vi "test_ssh.vi"(5 "Close?":bool=TRUE, 7 "Connection Info.":T2={"Remote"="10.8.2.13", "Username"="tvt", "Port (22)"=22}, 8 "error in (no error)":errorcluster, 9 "Delay Time (s)":dbl=10.0 format="%#_13g", 11 "cmd Box":string(combo)) -> (0 "error out":errorcluster, 2 "cmd string":string, 3 "remote log path":string)   [LabVIEW 2022 SP3]
uses:
  SSH Library/Connection Info..cluster.ctl
  SSH Library/Password..cluster.ctl
  <vilib>/Utility/error.llb/Trim Whitespace One-Sided.vi
  SSH Library/connect_password.vi
  SSH Library/LabSSH.lvlib
panel:
  out "Connection Name":string
  out "Method Response":string
  out "isSshConnected":bool
  in  "Password":T1={"Password"="TDDPc5kc4WnYcy"}
  out "Output":string
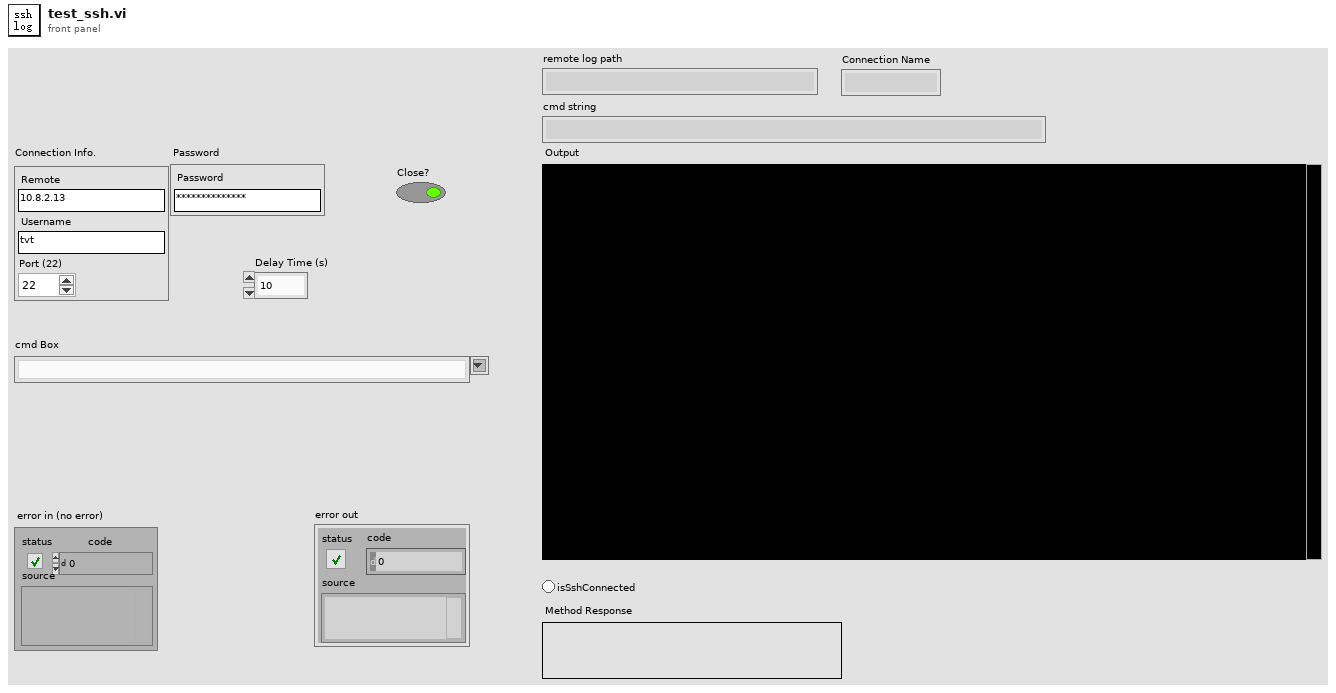
[diagram p1: front panel]
types:
  T1 = typedef "LabSSH.lvlib/Password..cluster.ctl" = cluster{"Password":string}
  T2 = typedef "LabSSH.lvlib/Connection Info..cluster.ctl" = cluster{"Remote":string, "Username":string, "Port (22)":i32}
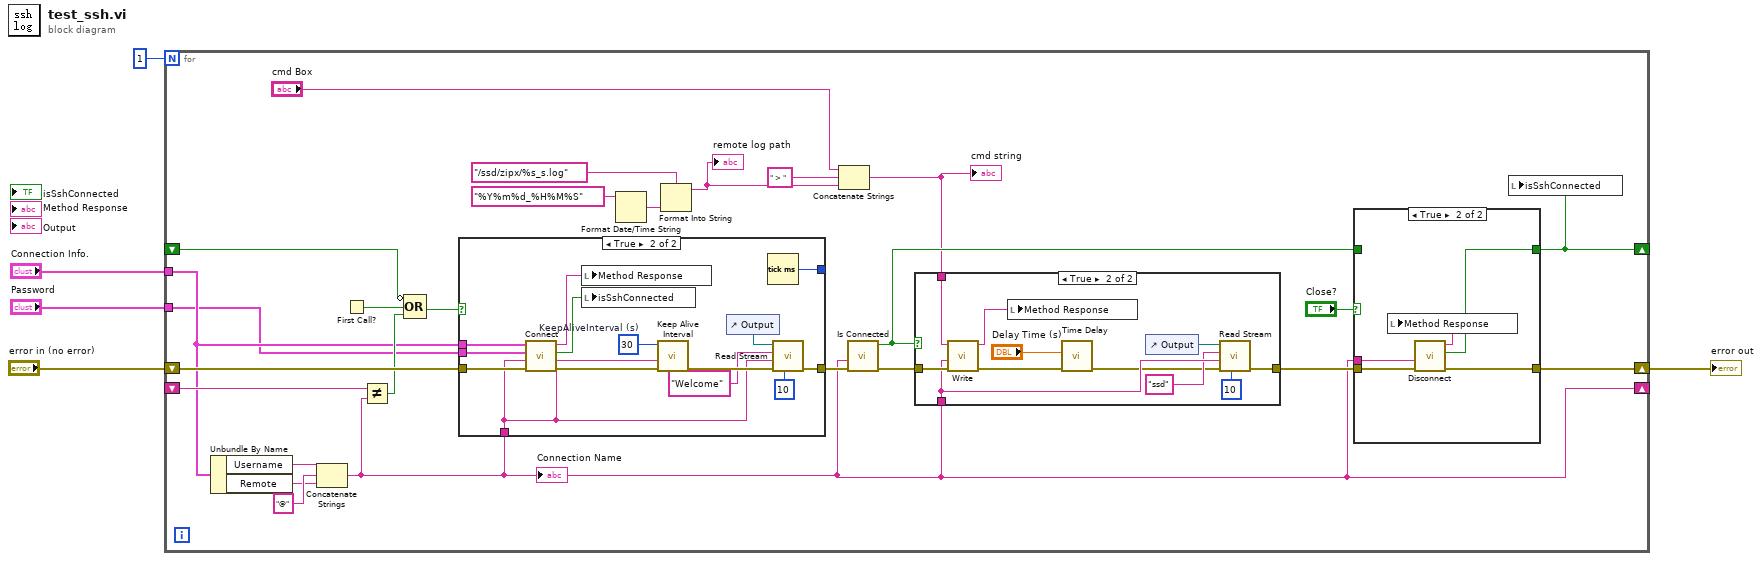
[diagram p0: block diagram]
diagram:
  n1 = for {
    N: 1 -> [_]
    shift-right: [w24] -> w1
    shift-left: "error in (no error)" -> [w28]
    shift-right: [w21] -> _
    shift-left: _ -> [w23]
    shift-right: [w16] -> _
    shift-left: _ -> [w17]
    tunnel: "Connection Info." -> [w14]
    tunnel: "Password" -> [w13]
    n2 = Unbundle By Name(w14) -> ("Username"=w22:string, "Remote"=w26:string)
    n3 = Concatenate Strings(w22, "@" ("string"), w26) -> (w21:string)
    "Connection Name" <- w21
    n4 = First Call?() -> (First Call?: T/F=w18:bool)
    n5 = Not Equal?(x=w23, y=w21) -> (x != y?=w20:bool)
    n6 = Compound Arithmetic op=OR(invert w17, w18, w20) -> (w19:bool)
    n7 = case shown="True" w19 {
      tunnel: w13 -> [_ w63]
      tunnel: [w51 w62] -> w31
      tunnel: w28 -> [w51 w56]
      tunnel: w14 -> [_ w55]
      tunnel: w21 -> [_ w54]
      tunnel: [_ w53] -> _
      frame False {
      }
      frame True {
        w57 = 30  # KeepAliveInterval (s)
        n8 = call-poly "Connect.vi"("error in (no error)"=w56, "Connection Name"=w54, "Password"=w63, "Connection Info."=w55) -> ("error out"=w58:errorcluster, "isSshConnected"=w61:bool, "Return String"=w60:string)  [unwired: 5 in]
        n9 = local write "Method Response"(w60) -> ()
        n10 = local write "isSshConnected"(w61) -> ()
        n11 = call "Keep Alive Interval.vi"("error in (no error)"=w58, "Connection Name"=w54, "KeepAliveInterval (s)"=w57) -> ("error out"=w59:errorcluster)  [unwired: 8 in]
        n12 = control-ref of="Output"() -> (w64:refnum<vi>)
        n13 = Tick Count (ms)() -> (millisecond timer value=w53:u32)
        n14 = call "Read Stream.vi"("Timout (s)"=10, "error in (no error)"=w59, "Connection Name"=w54, "Expected Response"="Welcome", "Output ref"=w64) -> ("error out"=w62:errorcluster)  [unwired: 6 in]
      }
    }
    n15 = Format Date/Time String(time format string (%c)="%Y%m%d_%H%M%S") -> (date/time string=w10:string)  [unwired: 2 in]
    n16 = Format Into String(format string="/ssd/zipx/%s_s.log", w10) -> (resulting string=w8:string)  [unwired: 2 in, 1 out]
    "remote log path" <- w8
    n17 = Concatenate Strings("cmd Box", " > " ("string"), w8) -> (w12:string)
    "cmd string" <- w12
    n18 = call "Is Connected.vi"("error in (no error)"=w31, "Connection Name"=w21) -> ("error out"=w30:errorcluster, "isSshConnected"=w15:bool)  [unwired: 8 in]
    n19 = case shown="True" w15 {
      tunnel: w30 -> [w39 w50]
      tunnel: [w39 w46] -> w29
      tunnel: w12 -> [_ w45]
      tunnel: w21 -> [_ w44]
      frame False {
      }
      frame True {
        n20 = call "Write.vi"("error in (no error)"=w50, "Connection Name"=w44, "Command"=w45) -> ("error out"=w42:errorcluster, "Return String"=w47:string)  [unwired: 7 in]
        n21 = local write "Method Response"(w47) -> ()
        n22 = call "Time Delay"("error in (no error)"=w42, "Delay Time (s)"="Delay Time (s)") -> ("error out"=w41:errorcluster)  [unwired: 9 in]
        n23 = control-ref of="Output"() -> (w49:refnum<vi>)
        n24 = call "Read Stream.vi"("Timout (s)"=10, "error in (no error)"=w41, "Connection Name"=w44, "Expected Response"="ssd", "Output ref"=w49) -> ("error out"=w46:errorcluster)  [unwired: 6 in]
      }
    }
    n25 = case shown="True" "Close?" {
      tunnel: w29 -> [w33 w38]
      tunnel: w21 -> [_ w37]
      tunnel: [w33 w35] -> w24
      tunnel: [w32 w34] -> w16
      tunnel: w15 -> [w32 _]
      frame False {
      }
      frame True {
        n26 = call "Disconnect.vi"("error in (no error)"=w38, "Connection Name"=w37) -> ("error out"=w35:errorcluster, "isSshConnected"=w34:bool, "Return String"=w36:string)  [unwired: 7 in]
        n27 = local write "Method Response"(w36) -> ()
      }
    }
    n28 = local write "isSshConnected"(w16) -> ()
  }
  "error out" <- w1
